vi "root_directory_list.vi"(5 "error in (no error)":errorcluster, 7 "文件夹":string(combo)) -> (1 "error out":errorcluster, 2 "目标路径":path, 3 "根路径":path)   [LabVIEW 2019]
doc: "*****注意：根路径的解析和本VI存放位置有关，需要自行修改*****\n可自行修改下拉列表，预设文件夹名称方便调用\n\n获取当前项目运行程序目录/根路径/设置的文件夹路径\n非法路径输出为默认根目录，需要注意"
panel:
  # "预设了下拉列表，可以快速选择\n非法路径结果输出根目录哈"
  # "获取当前的根目录\n需要根据实际情况修改"
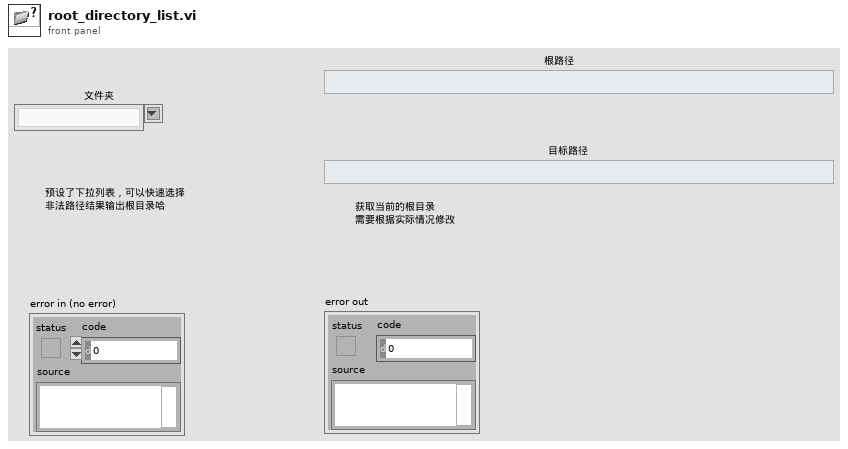
[diagram p1: front panel]
types:
  T1 = enum32{"invalid app kind", "Development System", "Run Time System", "Student Edition", "Embedded LabVIEW", "Evaluation", "Custom"}
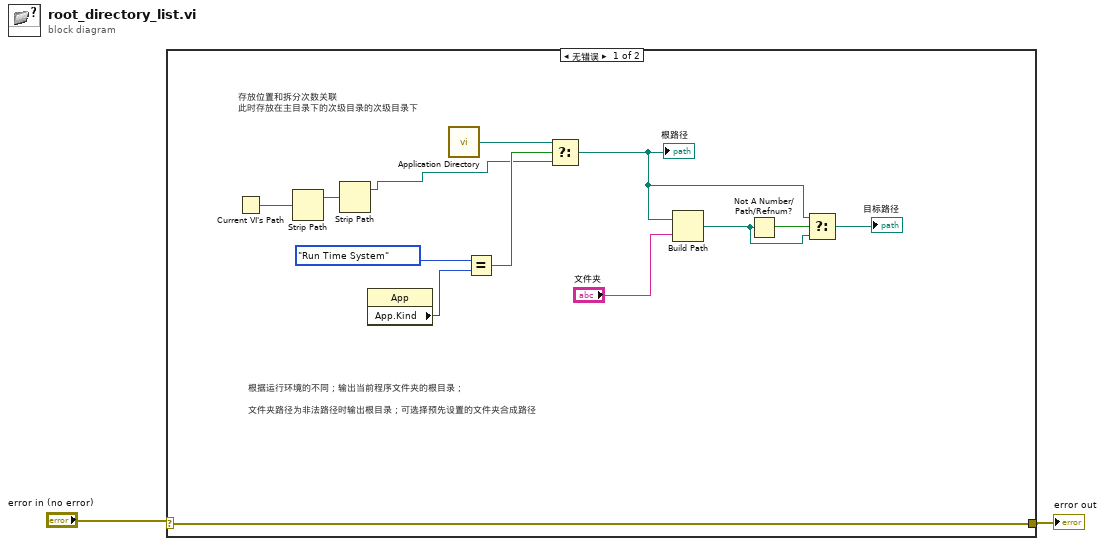
[diagram p0: block diagram]
diagram:
  n1 = case shown="无错误" "error in (no error)" {
    selector: "error in (no error)" -> [w4 w16]
    tunnel: [w4 w16] -> w1
    frame No Error {
      # "存放位置和拆分次数关联\n此时存放在主目录下的次级目录的次级目录下"
      # "根据运行环境的不同；输出当前程序文件夹的根目录；\n\n文件夹路径为非法路径时输出根目录；可选择预先设置的文件夹合成路径"
      n2 = Current VI's Path() -> (path=w14:path)
      n3 = Strip Path(path=w14) -> (stripped path=w5:path)  [unwired: 1 out]
      n4 = Strip Path(path=w5) -> (stripped path=w3:path)  [unwired: 1 out]
      n5 = property class="App"() -> ("App.Kind"=w13:T1)  [unwired: 2 in, 2 out]
      n6 = call <vilib>:"Application Directory.vi"() -> ("Application Directory"=w15:path)
      n7 = Equal?(x=T1."Run Time System", y=w13) -> (x = y?=w11:bool)
      n8 = Select(t=w15, s=w11, f=w3) -> (s? t:f=w7:path)
      "根路径" <- w7
      n9 = Build Path(base path=w7, name or relative path="文件夹") -> (appended path=w8:path)
      n10 = Not A Number/Path/Refnum?(number/path/refnum=w8) -> (NaN/Path/Refnum?=w9:bool)
      n11 = Select(t=w7, s=w9, f=w8) -> (s? t:f=→"目标路径":path)
    }
    frame Error {
    }
  }
  "error out" <- w1
